vi "Init Vecto.vi"(8 "error in (no error)":errorcluster, 11 "VolatusCore in":refnum<class "VolatusCore.lvclass">) -> (0 "error out":errorcluster, 3 "VolatusCore out":refnum<class "VolatusCore.lvclass">)   [LabVIEW 2020, in "Volatus.lvlib" / "VolatusCore.lvclass"]
uses:
  VolatusCore.lvclass
  lv-vecto/Vecto/Init Implementations.ctl
  lv-vecto/Vecto/EventLogHandler/EventLogHandler.lvclass
  lv-vecto/Vecto/Event Level.ctl
  VolatusCore.lvclass/VolatusCore.ctl
  VectoEventBridge/VectoEventBridge.lvclass
  C:/dev/lv20CE/relink/lv-vecto/Vecto/EventLogHandler/EventLogHandler.lvclass
  App/App.lvclass
  lv-vecto/Vecto/Vecto.lvlib
  lv-vecto/Vecto/Vecto/Vecto.lvclass
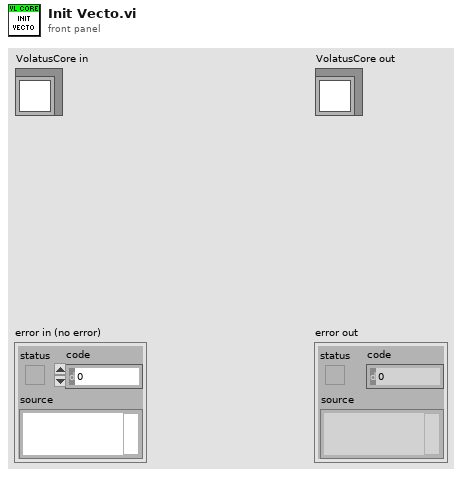
[diagram p1: front panel]
types:
  T1 = typedef "Vecto.lvlib/Event Level.ctl" = enum16{"Debug", "Info", "Warning", "Error"}
  T2 = typedef "Vecto.lvlib/Init Implementations.ctl" = cluster{"EventLogger":refnum<class "EventLogHandler.lvclass">}
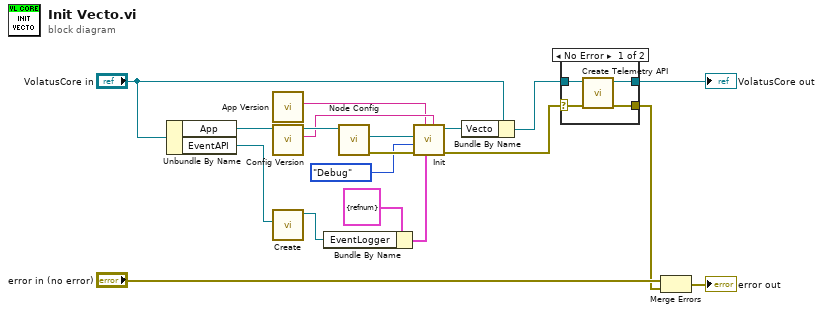
[diagram p0: block diagram]
diagram:
  n1 = Unbundle By Name("VolatusCore in") -> ("App"=w8:refnum<class "App.lvclass">, "EventAPI"=w7:refnum<class "EventAPI.lvclass">)
  n2 = call "App Version.vi"() -> ("App Version"=w11:string)  [unwired: 11 in]
  n3 = call "Config Version.vi"("App in"=w8) -> ("Cfg Version"=w12:string, "App out"=w13:refnum<class "App.lvclass">)  [unwired: 8 in, 1 out]
  n4 = call "Create.vi"("EventAPI"=w7) -> ("VectoEventBridge out"=w14:refnum<class "VectoEventBridge.lvclass">)  [unwired: 9 in, 1 out]
  n5 = Bundle By Name(cluster=T2 {"EventLogger"=refnum} ("Init Implementations"), "EventLogger"=w14) -> (w15:T2)
  n6 = call-dynamic "Node Config.vi"("App in"=w13) -> ("error out"=w18:errorcluster, "Node Config"=w17:refnum<class "Node Config.lvclass">)  [unwired: 8 in, 1 out]
  n7 = call "Init.vi"("Config Version"=w12, "Init Implementations"=w15, "App Version"=w11, "error in (no error)"=w18, "Minimum Event Level (Info)"=Event_Level."Debug", "Node"=w17) -> ("error out"=w3:errorcluster, "Vecto out"=w10:refnum<class "Vecto.lvclass">)  [unwired: 4 in]
  n8 = Bundle By Name(cluster="VolatusCore in", "Vecto"=w10) -> (w5:refnum<class "VolatusCore.lvclass">)
  n9 = case shown="No Error" w3 {
    selector: w3 -> [w21 w24]
    tunnel: w5 -> [w23 w25]
    tunnel: [w22 w25] -> w4
    tunnel: [w20 w24] -> w1
    frame No Error {
      n10 = call "Create Telemetry API.vi"("error in (no error)"=w21, "VolatusCore in"=w23) -> ("error out"=w20:errorcluster, "VolatusCore out"=w22:refnum<class "VolatusCore.lvclass">)  [unwired: 8 in]
    }
    frame Error {
    }
  }
  "VolatusCore out" <- w4
  n11 = Merge Errors("error in (no error)", w1) -> (→"error out":errorcluster)
